vi "Const bmp keyword.vi"() -> (3 "Const bmp keyword":string[](array[string]))   [LabVIEW 2018, in "Frame Analizer.lvclass"]
uses:
  Frame Analizer.lvclass
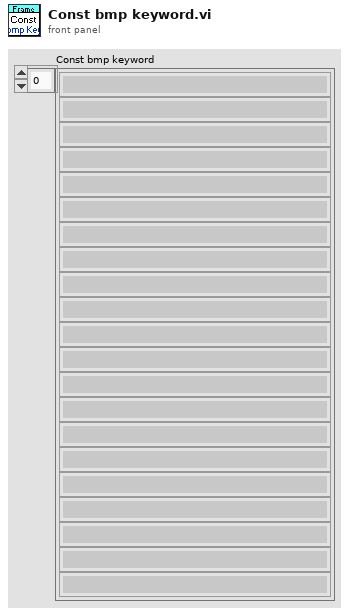
[diagram p1: front panel]
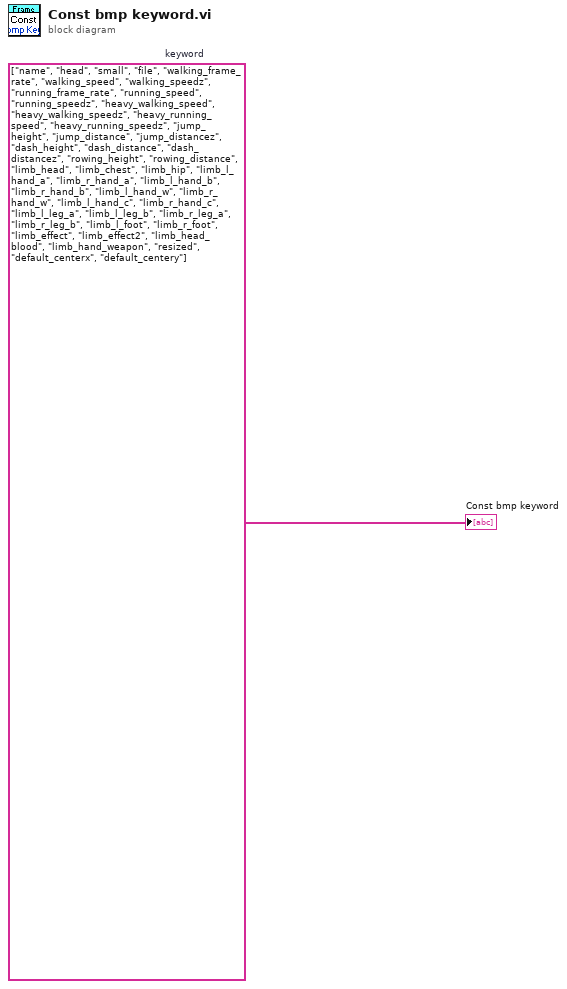
[diagram p0: block diagram]
diagram:
  w1 = string[] ["name", "head", "small", "file", "walking_frame_rate", "walking_speed", "walking_speedz", "running_frame_rate", "running_speed", "running_speedz", "heavy_walking_speed", "heavy_walking_speedz", "heavy_running_speed", "heavy_running_speedz", "jump_height", "jump_distance", "jump_distancez", "dash_height", "dash_distance", "dash_distancez", "rowing_height", "rowing_distance", "limb_head", "limb_chest", "limb_hip", "limb_l_hand_a", "limb_r_hand_a", "limb_l_hand_b", "limb_r_hand_b", "limb_l_hand_w", "limb_r_hand_w", "limb_l_hand_c", "limb_r_hand_c", "limb_l_leg_a", "limb_l_leg_b", "limb_r_leg_a", "limb_r_leg_b", "limb_l_foot", "limb_r_foot", "limb_effect", "limb_effect2", "limb_head_blood", "limb_hand_weapon", "resized", "default_centerx", "default_centery"]  # keyword
  "Const bmp keyword" <- w1
